vi "adder&subtractor.vi"() -> ()   [LabVIEW 2020]
panel:
  out "cout":bool
  out "s0":bool
  out "s1":bool
  out "s2":bool
  out "s3":bool
  in  "Enable":bool
  in  "b0":bool
  in  "b2":bool
  in  "b1":bool
  in  "b3":bool
  in  "a0":bool
  in  "a1":bool
  in  "a 2":bool
  in  "a3":bool
  # "First 4-bit number"
  # "Output"
  # "Second 4-bit number"
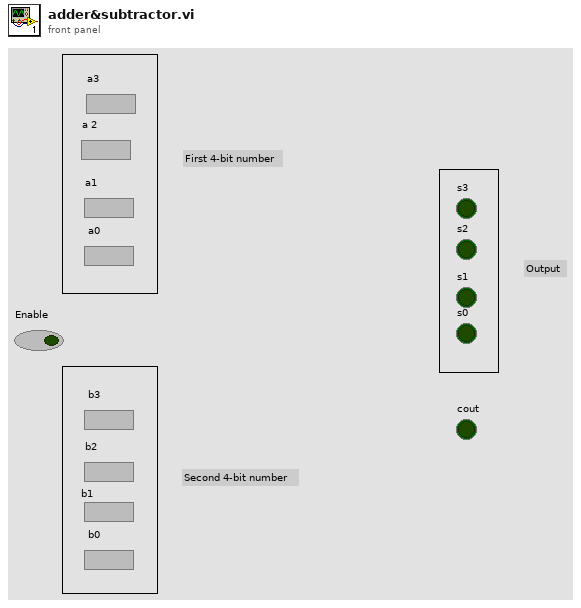
[diagram p1: front panel]
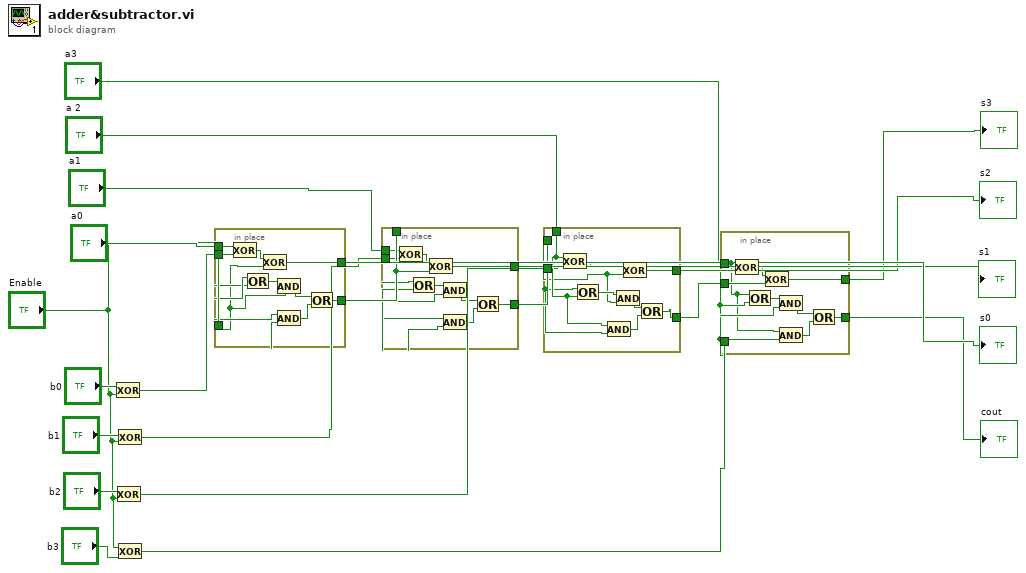
[diagram p0: block diagram]
diagram:
  n1 = Exclusive Or(1:"Enable", 2:"b0") -> (0:w3:bool)
  n2 = Exclusive Or(1:"Enable", 2:"b2") -> (0:w11:bool)
  n3 = Exclusive Or(1:"Enable", 2:"b1") -> (0:w15:bool)
  n4 = Exclusive Or(1:"b3", 2:"Enable") -> (0:w5:bool)
  n5 = in-place {
    in-place-border: "a0" -> [w27]
    in-place-border: [w25] -> w17
    in-place-border: [w24] -> w16
    in-place-border: w3 -> [w23]
    in-place-border: "Enable" -> [w22]
    n6 = Exclusive Or(1:w23, 2:w27) -> (0:w30:bool)
    n7 = Or(x=w27, y=w23) -> (x .or. y?=w29:bool)
    n8 = Exclusive Or(1:w22, 2:w30) -> (0:w25:bool)
    n9 = And(x=w29, y=w22) -> (x .and. y?=w28:bool)
    n10 = And(x=w27, y=w23) -> (x .and. y?=w26:bool)
    n11 = Or(x=w28, y=w26) -> (x .or. y?=w24:bool)
  }
  "s0" <- w17
  n12 = in-place {
    in-place-border: w16 -> [w35]
    in-place-border: w15 -> [w34]
    in-place-border: "a1" -> [w33]
    in-place-border: [w32] -> w13
    in-place-border: [w31] -> w9
    n13 = Exclusive Or(1:w34, 2:w33) -> (0:w39:bool)
    n14 = Or(x=w33, y=w34) -> (x .or. y?=w38:bool)
    n15 = Exclusive Or(1:w35, 2:w39) -> (0:w32:bool)
    n16 = And(x=w38, y=w35) -> (x .and. y?=w37:bool)
    n17 = And(x=w33, y=w34) -> (x .and. y?=w36:bool)
    n18 = Or(x=w37, y=w36) -> (x .or. y?=w31:bool)
  }
  "s1" <- w13
  n19 = in-place {
    in-place-border: "a 2" -> [w44]
    in-place-border: w11 -> [w43]
    in-place-border: [w42] -> w10
    in-place-border: w9 -> [w41]
    in-place-border: [w40] -> w6
    n20 = Exclusive Or(1:w43, 2:w44) -> (0:w48:bool)
    n21 = Or(x=w43, y=w44) -> (x .or. y?=w47:bool)
    n22 = And(x=w44, y=w43) -> (x .and. y?=w45:bool)
    n23 = And(x=w47, y=w41) -> (x .and. y?=w46:bool)
    n24 = Exclusive Or(1:w41, 2:w48) -> (0:w42:bool)
    n25 = Or(x=w46, y=w45) -> (x .or. y?=w40:bool)
  }
  "s2" <- w10
  n26 = in-place {
    in-place-border: [w53] -> w8
    in-place-border: [w52] -> w7
    in-place-border: w6 -> [w51]
    in-place-border: w5 -> [w50]
    in-place-border: "a3" -> [w49]
    n27 = Exclusive Or(1:w50, 2:w49) -> (0:w57:bool)
    n28 = Or(x=w49, y=w50) -> (x .or. y?=w56:bool)
    n29 = Exclusive Or(1:w51, 2:w57) -> (0:w53:bool)
    n30 = And(x=w56, y=w51) -> (x .and. y?=w55:bool)
    n31 = And(x=w49, y=w50) -> (x .and. y?=w54:bool)
    n32 = Or(x=w55, y=w54) -> (x .or. y?=w52:bool)
  }
  "s3" <- w8
  "cout" <- w7
